vi "_Test_Read_RDB_Objs.vi"() -> ()   [LabVIEW 2023]
uses:
  RDB/RDB Object.ctl
  RDB/RDB Player Object.ctl
  RDB/RDB Reference.ctl
  <vilib>/xnet/xnet.llb/XNET Frame FlexRay.ctl
  <vilib>/xnet/xnet.llb/XNET Frame Type FlexRay.ctl
  <vilib>/Utility/xml.llb/Read From XML File(string).vi
  RDB/RDB.lvlib
panel:
  out "RDB Reference":T1 {"RDB Data"."payload" format="%x"; "RDB Data"."timestamp" format="%<%.7X\n%x>T"; "RDB Data"."type" items=["FlexRay Data"=32, "FlexRay Null"=33, "FlexRay Symbol"=34, "Log Trigger"=225, "Start Trigger"=226]; "RDB Data"."cycle count" max=63 step=1}
  out "value":T4[](array[typedef])
  in  "XML File Path":path=path "C:/Debug/Receive.xml"
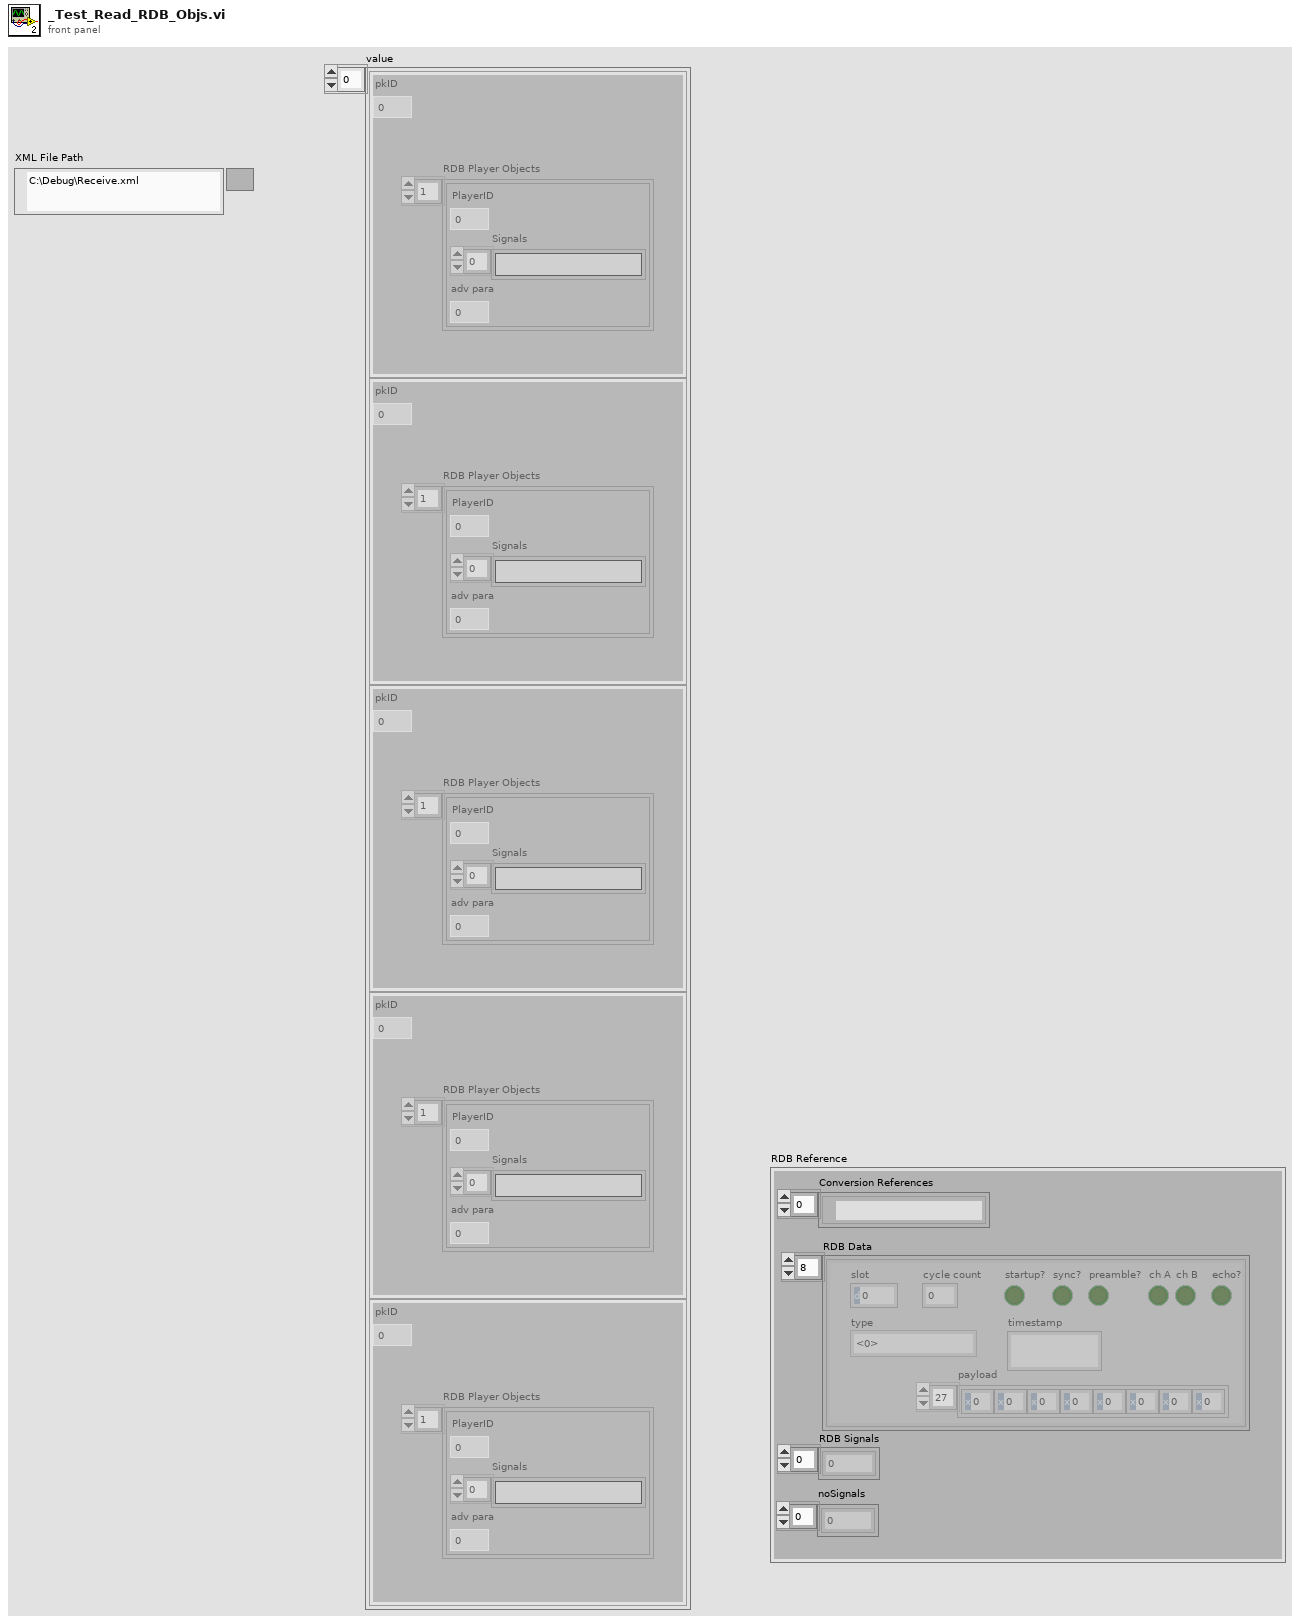
[diagram p1: front panel]
types:
  T1 = typedef "RDB.lvlib/RDB Reference.ctl" = cluster{"Conversion References":refnum<k21>[], "RDB Data":T2[], "RDB Signals":dbl[], "noSignals":i32[]}
  T2 = typedef "XNET Frame FlexRay.ctl" = cluster{"timestamp":timestamp, "payload":u8[], "slot":u16, "type":T3, "cycle count":u8, "startup?":bool, "sync?":bool, "preamble?":bool, "ch A":bool, "ch B":bool, "echo?":bool}
  T3 = typedef "XNET Frame Type FlexRay.ctl" = u8
  T4 = typedef "RDB.lvlib/RDB Object.ctl" = cluster{"pkID":i32, "RDB Player Objects":T5[]}
  T5 = typedef "RDB.lvlib/RDB Player Object.ctl" = cluster{"PlayerID":i32, "Signals":string[], "adv para":i32}
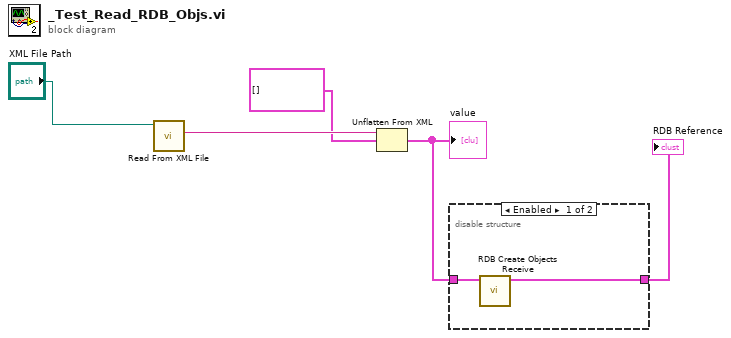
[diagram p0: block diagram]
diagram:
  n1 = call-poly <vilib>:"Read From XML File.vi"("XML File Path"="XML File Path") -> ("XML Elements"=w5:string)  [unwired: 8 in, 2 out]
  n2 = Unflatten From XML(xml string=w5, type=T4[] []) -> (value=w2:T4[])  [unwired: 1 in, 1 out]
  "value" <- w2
  n3 = disable-structure shown="Enabled" {
    disable-tunnel: w2 -> [w7 _]
    disable-tunnel: [w6 _] -> w1
    frame Enabled {
      n4 = call "RDB Create Objects Receive.vi"("RDB Data Receive"=w7) -> ("RDB Reference"=w6:T1)  [unwired: 9 in, 1 out]
    }
    frame Disabled {
    }
  }
  "RDB Reference" <- w1
